vi "状态显示参数.vi"() -> ()   [LabVIEW 2013]
panel:
  in  "状态显示参数":T1 {"标准转速" format="%0.1f rpm"; "DEH指令值" scale=0.0..100.0; "LVDT2信号采样百分比" scale=0.0..100.0; "LVDT1信号采样百分比" scale=0.0..100.0}
  # "转速反馈"
  # "LVDT 1"
  # "LVDT 2"
  # "阀门输出"
  # "伺服输出使能"
  # "DEH"
  # "转速标定"
  # "输出通道状态"
  # "伺服阀输出电流"
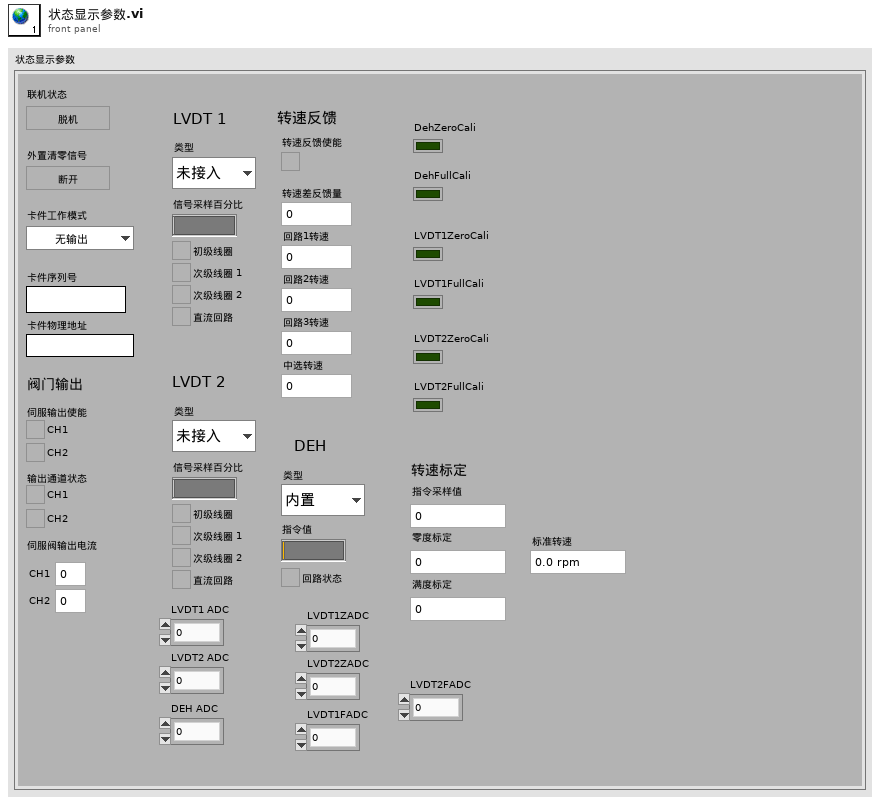
[diagram p1: front panel]
types:
  T1 = cluster{"联机状态":bool, "外置清零信号":bool, "卡件工作模式":enum16{"无输出", "正常工作", "阀门常开", "阀门常闭"}, "卡件序列号":string, "卡件物理地址":string, "伺服阀输出电流CH1":dbl, "输出通道状态CH1":bool, "伺服阀输出电流CH2":dbl, "输出通道状态CH2":bool, "伺服输出使能CH1 ":bool, "伺服输出使能CH2":bool, "LVDT1类型":enum16{"未接入", "直流", "交流"}, "LVDT1直流回路":bool, "LVDT1次级线圈 2":bool, "LVDT1次级线圈 1":bool, "LVDT1初级线圈":bool, "LVDT2类型":enum16{"未接入", "直流", "交流"}, "LVDT2直流回路":bool, "LVDT2次级线圈 2":bool, "LVDT2次级线圈 1":bool, "LVDT2初级线圈":bool, "DEH回路状态":bool, "DEH类型":enum16{"内置", "外接"}, "转速反馈使能":bool, "LVDT1信号采样百分比":dbl, "LVDT2信号采样百分比":dbl, "DEH指令值":u8, "转速差反馈量":dbl, "回路1转速":dbl, "回路2转速":dbl, "回路3转速":dbl, "中选转速":dbl, "LVDT1 ADC":i16, "LVDT2 ADC":i16, "DEH ADC":i16, "LVDT1ZADC":i16, "LVDT2ZADC":i16, "LVDT1FADC":i16, "LVDT2FADC":i16, "DehZeroCali":bool, "DehFullCali":bool, "LVDT1ZeroCali":bool, "LVDT1FullCali":bool, "LVDT2ZeroCali":bool, "LVDT2FullCali":bool, "转速零度标定":i16, "转速满度标定":i16, "转速指令采样值":i16, "标准转速":dbl}
diagram:
